vi "Period Counter.vi"() -> ()   [LabVIEW 2015]
uses:
  <vilib>/DAQmx/read.llb/DAQmx Read (Counter 1D DBL 1Chan NSamp).vi
  <vilib>/Analysis/baseanly.llb/Mean (DBL).vi
  <vilib>/DAQmx/create/channels.llb/DAQmx Create Channel (CI-Period).vi
  <vilib>/DAQmx/configure/timing.llb/DAQmx Timing (Implicit).vi
  <vilib>/DAQmx/miscellaneous.llb/DAQmx Fill In Error Info.vi
  <vilib>/Analysis/NI_AALBase.lvlib
  <resource>/objmgr/daqmx.rc
panel:
  out "divisor":u32=4
  out "Period (ms)":dbl format="%g ms"
  in  "Stop":bool
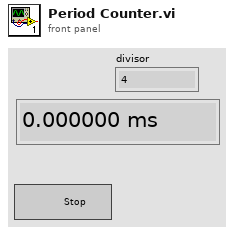
[diagram p1: front panel]
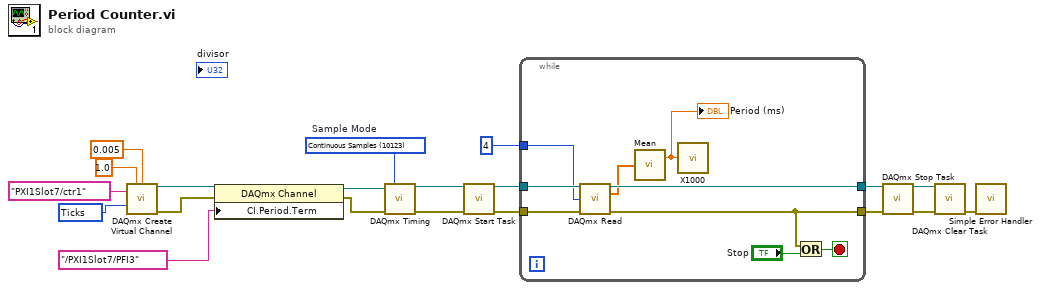
[diagram p0: block diagram]
diagram:
  w1 = 10304 items=["Seconds"=10364, "Ticks"=10304, "From Custom Scale"=10065] ("units")
  w19 = 10123 items=["Finite Samples"=10178, "Continuous Samples"=10123, "Hardware Timed Single Point"=12522]  # Sample Mode
  n1 = call-poly <vilib>:"DAQmx Create Virtual Channel.vi"("maximum value"=1.0, "minimum value"=0.005, "counter"=tag "PXI1Slot7/ctr1", "units"=w1) -> ("task out"=w5:refnum<k21>, "error out"=w3:errorcluster)  [unwired: 10 in]
  n2 = property class="DAQmx Channel"(reference=w5, error in=w3, "CI.Period.Term"=tag "/PXI1Slot7/PFI3" ("Period Input Terminal")) -> (reference out=w4:refnum<k21>, error out=w2:errorcluster)
  n3 = call-poly <vilib>:"DAQmx Timing.vi"("task/channels in"=w4, "sample mode"=w19, "error in"=w2) -> ("task out"=w12:refnum<k21>, "error out"=w11:errorcluster)  [unwired: 11 in]
  n4 = call <vilib>:"DAQmx Start Task.vi"("task/channels in"=w12, "error in"=w11) -> ("task out"=w13:refnum<k21>, "error out"=w14:errorcluster)  [unwired: 12 in]
  n5 = while {
    tunnel: w13 -> [w29]
    tunnel: w14 -> [w28]
    tunnel: [w24] -> w18
    tunnel: [w26] -> w17
    tunnel: 4 -> [w23]
    stop <- w27 stop-if-true
    n6 = call-poly <vilib>:"DAQmx Read.vi"("task/channels in"=w29, "number of samples per channel"=w23, "error in"=w28) -> ("task out"=w26:refnum<k21>, "data"=w22:dbl[], "error out"=w24:errorcluster)  [unwired: 10 in]
    n7 = call-poly <vilib>:"Mean.vi"("X"=w22) -> ("mean"=w21:dbl)  [unwired: 1 out]
    "Period (ms)" <- w21
    n8 = call "X1000.vi"("X"=w21) -> ()  [unwired: 1 out]
    n9 = Or(x=w24, y="Stop") -> (x .or. y?=w27:bool)
  }
  n10 = call <vilib>:"DAQmx Stop Task.vi"("task/channels in"=w17, "error in"=w18) -> ("task out"=w15:refnum<k21>, "error out"=w16:errorcluster)  [unwired: 12 in]
  n11 = call <vilib>:"DAQmx Clear Task.vi"("task in"=w15, "error in"=w16) -> ("error out"=w10:errorcluster)  [unwired: 13 in]
  n12 = call <vilib>:"Simple Error Handler.vi"("error in (no error)"=w10) -> ()  [unwired: 4 in, 5 out]
